vi "Linear_fit.vi"(4 "Point selector":cluster{"Y":dbl, "X":dbl, "switch":bool}[](array[cluster]) {"X" format="%.2f"; "Y" format="%.2f"}, 5 "Input X array":dbl[](array[numeric]) format="%.3f", 7 "Input Y array":dbl[](array[numeric]) format="%.4f") -> (0 "Calib const":string[][](array[string]), 1 "Calibration plot":cluster{cluster{dbl, dbl}[]}[](graph), 2 "Coefficients":dbl[](array[numeric]) format="%.2f", 3 "Point selector":cluster{"Y":dbl, "X":dbl, "switch":bool}[](array[cluster]) {"X" format="%.2f"; "Y" format="%.2f"})   [LabVIEW 2010]
uses:
  <vilib>/Analysis/NI_AALPro.lvlib
  <vilib>/Analysis/NI_AALBase.lvlib
panel:
  in  "Type":cluster{"Y":dbl, "X":dbl, "switch":bool}={"Y"=10.144154930121, "X"=9.20412, "switch"=FALSE} {"X" format="%.2f"; "Y" format="%.2f"}
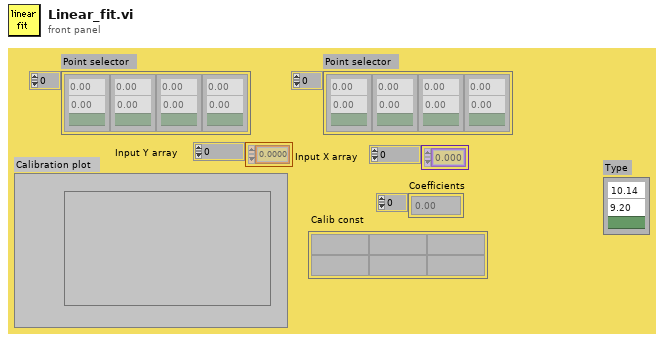
[diagram p1: front panel]
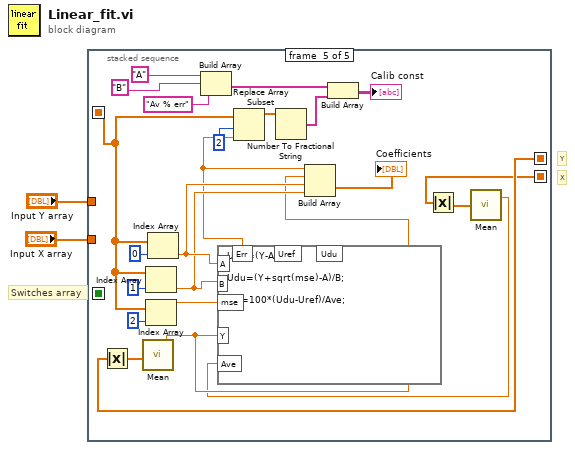
[diagram p0: block diagram]
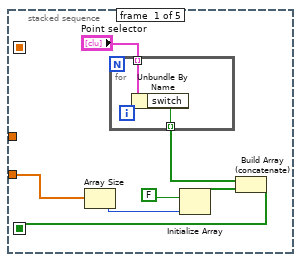
[diagram p2: hidden frame]
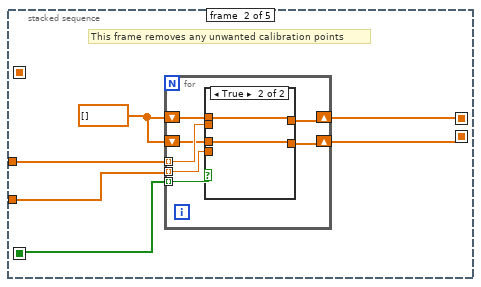
[diagram p3: hidden frame]
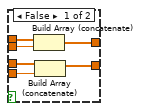
[diagram p4: hidden frame]
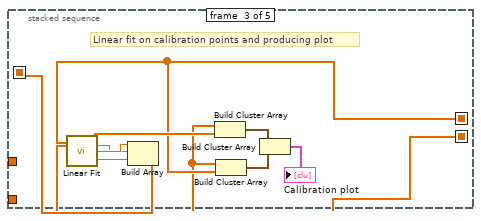
[diagram p5: hidden frame]
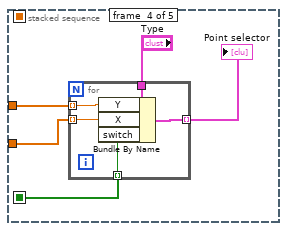
[diagram p6: hidden frame]
diagram:
  # "Switches array"
  # "X"
  # "Y"
  n1 = stacked-sequence {
    seq-local: [_ w17 _ _ _] -> [_ _ w34 _ w62]
    seq-local: [_ w16 _ _ _] -> [_ _ w33 _ w55]
    seq-local: [w7 _ _ _ _] -> [_ w13 _ w44 _]
    seq-local: [_ _ w35 _ _] -> [_ _ _ _ w70]
    tunnel: "Input X array" -> [w3 w14 _ w45 _]
    tunnel: "Input Y array" -> [_ w15 _ w46 _]
    frame #0 {
      n2 = Array Size(array=w3) -> (size(s)=w5:i32)
      n3 = for {
        tunnel: "Point selector" -> [w11] mode=indexing
        tunnel: [w10] -> w8 mode=indexing
        n4 = Unbundle By Name(w11) -> ("switch"=w10:bool)
      }
      n5 = Initialize Array(FALSE, w5) -> (w4:bool[])
      n6 = Build Array (concatenate)(w8, w4) -> (w7:bool[])
    }
    frame #1 {
      w12 = dbl[] []
      # "This frame removes any unwanted calibration points"
      n7 = for {
        shift-right: [w18] -> w16
        shift-left: w12 -> [w20]
        shift-right: [w19] -> w17
        shift-left: w12 -> [w21]
        tunnel: w13 -> [w22] mode=indexing
        tunnel: w14 -> [w23] mode=indexing
        tunnel: w15 -> [w24] mode=indexing
        n8 = case shown="True" w22 {
          tunnel: [w25 w31] -> w18
          tunnel: [w26 w32] -> w19
          tunnel: w20 -> [w27 w31]
          tunnel: w21 -> [w28 w32]
          tunnel: w23 -> [w29 _]
          tunnel: w24 -> [w30 _]
          frame False {
            n9 = Build Array (concatenate)(w28, w30) -> (w26:dbl[])
            n10 = Build Array (concatenate)(w27, w29) -> (w25:dbl[])
          }
          frame True {
          }
        }
      }
    }
    frame #2 {
      # "Linear fit on calibration points and producing plot"
      n11 = call <vilib>:"Linear Fit.vi"("Y"=w34, "X"=w33) -> ("Best Linear Fit"=w36:dbl[], "slope"=w37:dbl, "intercept"=w38:dbl, "residue"=w39:dbl)  [unwired: 4 in, 6 out]
      n12 = Build Array(w38, w37, w39) -> (w35:dbl[])
      n13 = Build Cluster Array(w33, w36) -> (w42:cluster{dbl, "Numeric":dbl}[])
      n14 = Build Cluster Array(w33, w34) -> (w41:cluster{dbl, dbl}[])
      n15 = Build Cluster Array(w42, w41) -> (→"Calibration plot":cluster{cluster{dbl, "Numeric":dbl}[]}[])
    }
    frame #3 {
      n16 = for {
        tunnel: "Type" -> [w52]
        tunnel: w46 -> [w51] mode=indexing
        tunnel: w45 -> [w50] mode=indexing
        tunnel: w44 -> [w49] mode=indexing
        tunnel: [w48] -> w43 mode=indexing
        n17 = Bundle By Name(cluster=w52, "Y"=w51, "X"=w50, "switch"=w49) -> (w48:cluster{"Y":dbl, "X":dbl, "switch":bool})
      }
      "Point selector" <- w43
    }
    frame #4 {
      n18 = Absolute Value(x=w62) -> (abs(x)=w56:dbl[])
      n19 = call <vilib>:"Mean.vi"("X"=w56) -> ("mean"=w57:dbl)  [unwired: 1 out]
      n20 = Index Array(array=w70, index=1) -> (element=w60:dbl)
      n21 = Index Array(array=w70, index=2) -> (element=w72:dbl)
      n22 = Index Array(array=w70, index=0) -> (element=w61:dbl)
      n23 = Build Array("A", "B", "Av % err") -> (w64:string[])
      n24 = Absolute Value(x=w55) -> (abs(x)=w54:dbl[])
      n25 = call <vilib>:"Mean.vi"("X"=w54) -> ("mean"=w53:dbl)  [unwired: 1 out]
      n26 = formula code="Uref=(Y-A)/B;\n\nUdu=(Y+sqrt(mse)-A)/B;\n\nErr=100*(Udu-Uref)/Ave;"("A"=w61, "B"=w60, "mse"=w72, "Y"=w57, "Ave"=w53) -> ("Err"=w58:dbl)  [unwired: 2 out]
      n27 = Replace Array Subset(array=w70, new element=w58, index=2) -> (w66:dbl[])
      n28 = Number To Fractional String(number=w66) -> (F-format string=w65:string[])  [unwired: 3 out]
      n29 = Build Array(w58, w57, w61, w60) -> (→"Coefficients":dbl[])
      n30 = Build Array(w64, w65) -> (→"Calib const":string[][])
    }
  }
